vi "Robotics Environment Simulator.vi"() -> ()   [LabVIEW 2013]
doc: "This VI starts and stops the environment simulator and serves as the master VI for your simulation code. Open and run this VI to display the environment simulator, or open the block diagram to view or modify simulation code."
uses:
  <vilib>/robotics/Simulator/Engine/ctl/Step Mode.ctl
  <vilib>/robotics/Simulator/Engine/ctl/DeviceID.ctl
  <vilib>/robotics/Simulator/Engine/ctl/Robot Component ID.ctl
  <resource>/robotics/simulator/Utility/ModelBuilder/Utilities/3DController/Public/ActionType.ctl
  <resource>/robotics/simulator/Utility/ModelBuilder/Utilities/3DController/3DController.lvclass
  <instrlib>/Hitec HS400 Series/HAIOL/Hitec HS400 Series.lvclass
  <vilib>/Analysis/7linalg.llb/Real Transpose Matrix.vi
  <vilib>/Analysis/baseanly.llb/A x Vector.vi
  <vilib>/Analysis/baseanly.llb/Real A x B.vi
  <vilib>/Analysis/_algsub.llb/Real Vector Norm.vi
  <vilib>/Analysis/baseanly.llb/Outer Product.vi
  <vilib>/Analysis/baseanly.llb/Real Outer Product.vi
  <vilib>/robotics/Kinematics/Create Lie Group Matrix.vi
  <vilib>/robotics/Simulator/Interface/Simulator References/Get Robot Component Reference.vi
  <vilib>/robotics/Simulator/Interface/Simulator References/Get 3D Visual Scene Reference.vi
  <vilib>/Analysis/baseanly.llb/Real Inverse Matrix.vi
  <vilib>/Analysis/7linalg.llb/Create Special Matrix.vi
  <vilib>/Analysis/7linalg.llb/Create Special Real Matrix.vi
  <vilib>/Analysis/Matrix/Numeric/Multiply/Multiply.vi
  <vilib>/Analysis/Matrix/Numeric/Multiply/Multiply - RM,R.vi
  <vilib>/Analysis/Matrix/Numeric/Multiply/Multiply - R,RM.vi
  <vilib>/Analysis/Matrix/Numeric/Add/Add.vi
  <vilib>/Analysis/Matrix/Numeric/Add/Add - RM,RM.vi
  <vilib>/robotics/Simulator/NI_Robotics_Simulator.lvlib
  <instrlib>/Hitec HS400 Series/HAIOL/Simulator/Hitec HS400 Series Simulator.lvclass
  <resource>/objmgr/LVODE.rc
  <vilib>/Analysis/NI_AALPro.lvlib
  <vilib>/Analysis/NI_AALBase.lvlib
  <vilib>/robotics/Kinematics/NI_Kinematics.lvlib
panel:
  out "p":dbl[](array[numeric])
  out "3D Picture":refnum<vi>(3d-picture)
  out "Waveform Chart":dbl(graph)
  out "exist":bool
  out "exit":bool
  out "target pos":dbl[](array[numeric])
  out "joints":dbl[](array[numeric])
  in  "manifest filename":string="Robotics Environment Simulator.xml"
  in  "stop":bool
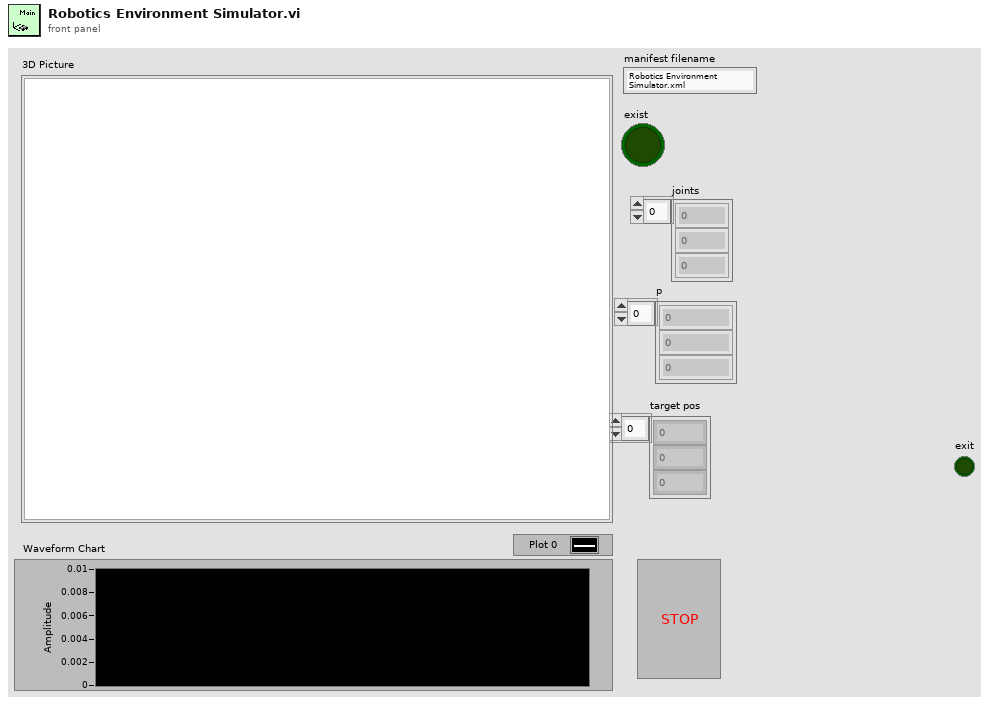
[diagram p1: front panel]
types:
  T1 = typedef "NI_Robotics_Simulator.lvlib/Step Mode.ctl" = u16
  T2 = typedef "NI_Robotics_Simulator.lvlib/DeviceID.ctl" = cluster{"robot ID":string, "sensor/actuator ID":string}
  T3 = typedef "NI_Robotics_Simulator.lvlib/Robot Component ID.ctl" = cluster{"robot ID":string, "component ID":string}
  T4 = typedef "NI_Robotics_Model_Builder.lvlib/3DController.lvclass/ActionType.ctl" = enum16{"None", "Trans_X", "Trans_Y", "Trans_Z", "Rot_X", "Rot_Y", "Rot_Z"}
  T5 = cluster{"Position[0]":sgl, "Position[1]":sgl, "Position[2]":sgl}
  T6 = typedef "NI_Matrix.lvlib/RealMatrix.ctl" = dbl[][]
  T7 = typedef "LVPoint32TypeDef.ctl" = cluster{"Horizontal":i32, "Vertical":i32}
  T8 = typedef "LV3DPointTypeDef.ctl" = cluster{"X":sgl, "Y":sgl, "Z":sgl}
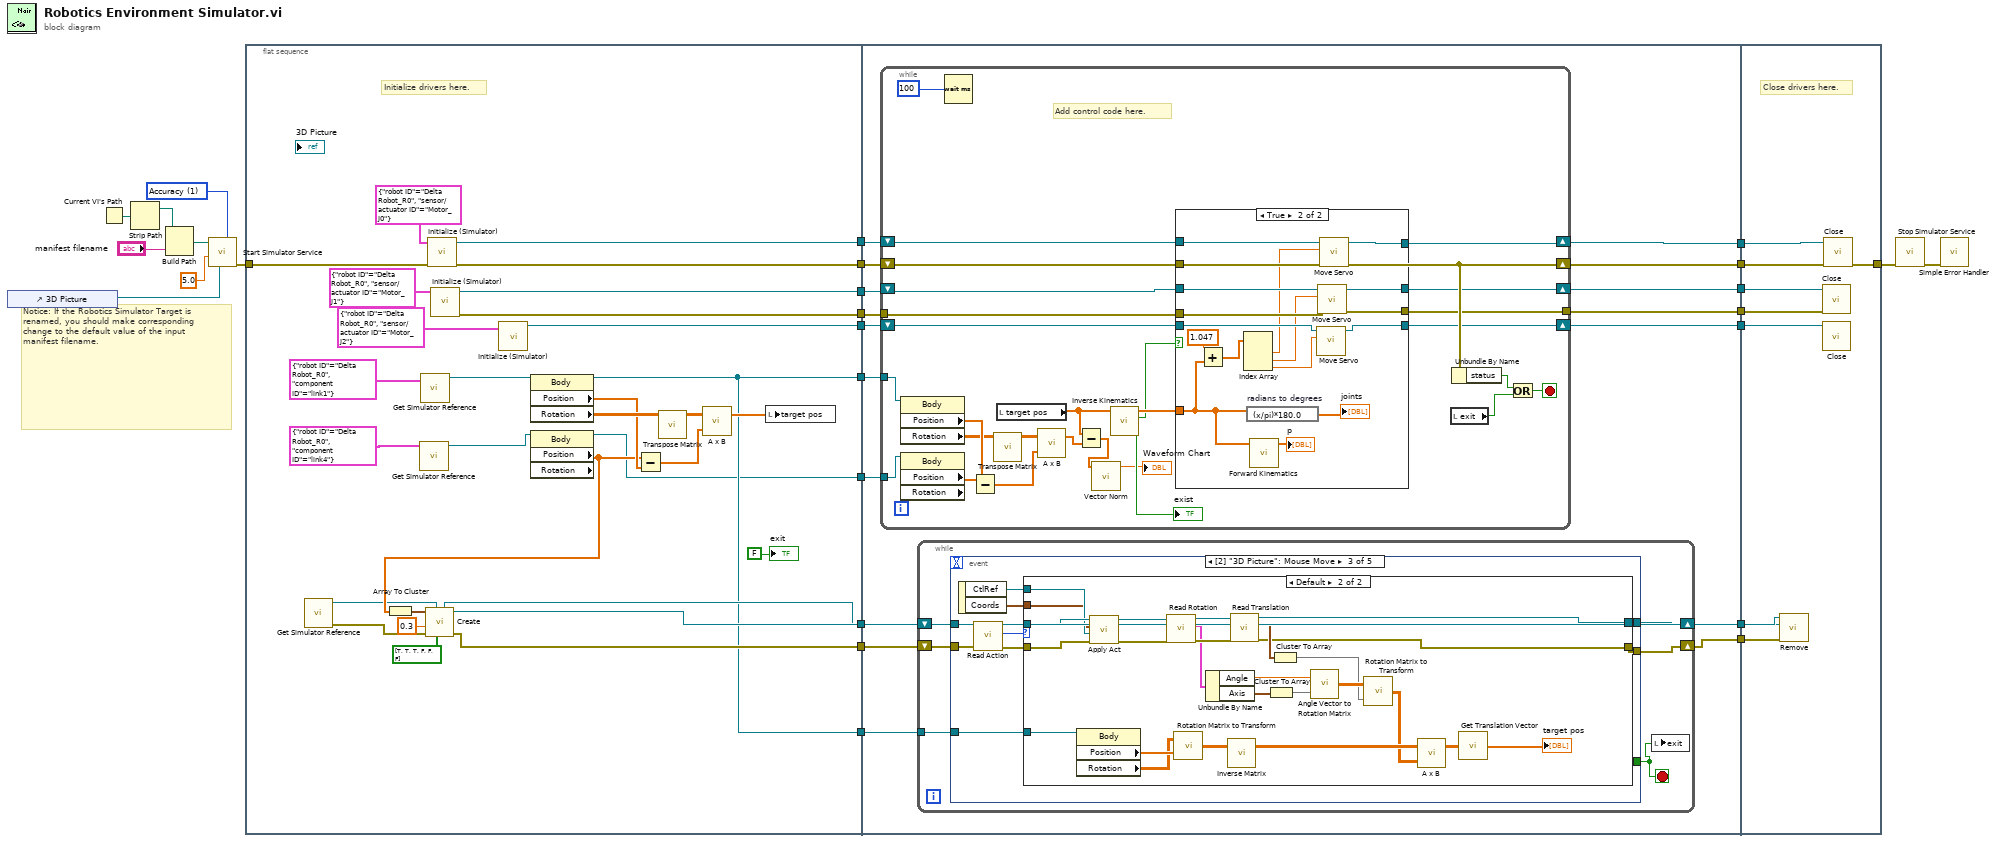
[diagram p0: block diagram]
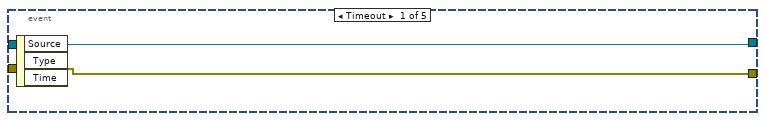
[diagram p2: hidden frame]
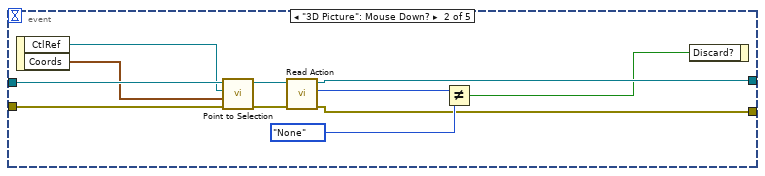
[diagram p3: hidden frame]
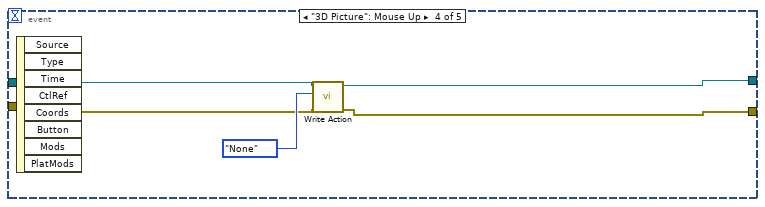
[diagram p5: hidden frame]
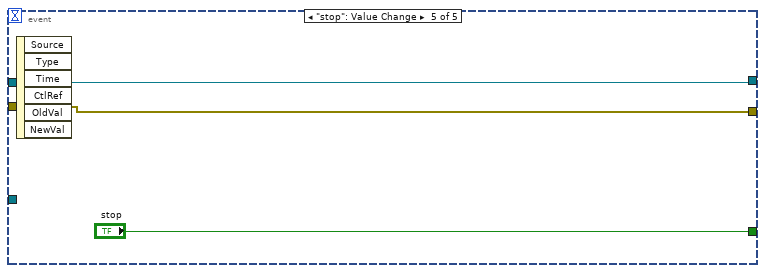
[diagram p6: hidden frame]
diagram:
  w13 = T1 1 items=["Performance", "Accuracy"] ("step mode")
  # "Notice: If the Robotics Simulator Target is renamed, you should make corresponding change to the default value of the input manifest filename."
  n1 = control-ref of="3D Picture"() -> (w1:refnum<vi>)
  n2 = Current VI's Path() -> (path=w27:path)
  n3 = Strip Path(path=w27) -> (stripped path=w26:path)  [unwired: 1 out]
  n4 = Build Path(base path=w26, name or relative path="manifest filename") -> (appended path=w25:path)
  n5 = call <vilib>:"Start Simulator Service.vi"("step mode"=w13, "3D picture refnum"=w1, "step size (ms)"=5.0 ("stepsize(ms)"), "manifest file"=w25) -> ("error out"=w22:errorcluster)  [unwired: 7 in]
  n6 = flat-sequence {
    tunnel: w22 -> [w57]
    tunnel: [w57] -> w21
    tunnel: [w56] -> w19
    tunnel: [w54] -> w17
    tunnel: [w53] -> w16
    tunnel: [w38] -> w12
    tunnel: [w37] -> w11
    tunnel: [w31] -> w10
    tunnel: [w34] -> w9
    tunnel: [w32] -> w5
    tunnel: [w31] -> w3
    tunnel: [w30] -> w2
    tunnel: w21 -> [w75]
    tunnel: [w76] -> w20
    tunnel: w19 -> [w74]
    tunnel: [w73] -> w18
    tunnel: w17 -> [w72]
    tunnel: w16 -> [w71]
    tunnel: [w70] -> w15
    tunnel: [w69] -> w14
    tunnel: w12 -> [w68]
    tunnel: w11 -> [w67]
    tunnel: w10 -> [w66]
    tunnel: w9 -> [w65]
    tunnel: [w64] -> w8
    tunnel: [w63] -> w7
    tunnel: [w62] -> w6
    tunnel: w5 -> [w61]
    tunnel: [w61] -> w4
    tunnel: w3 -> [w60]
    tunnel: w2 -> [w59]
    tunnel: [w194] -> w28
    tunnel: w20 -> [w196]
    tunnel: w18 -> [w195]
    tunnel: w15 -> [w193]
    tunnel: w14 -> [w192]
    tunnel: w8 -> [w191]
    tunnel: w7 -> [w190]
    tunnel: w6 -> [w189]
    tunnel: w4 -> [w188]
    frame #0 {
      # "Initialize drivers here."
      n7 = call-poly <vilib>:"Get Simulator Reference.vi"() -> ("error out"=w40:errorcluster, "scene ref"=w41:refnum<vi>)  [unwired: 10 in]
      n8 = call-poly <vilib>:"Get Simulator Reference.vi"("robot component ID"=T3 {"robot ID"="Delta Robot_R0", "component ID"="link4"}) -> ("component ref"=w44:refnum<k20>)  [unwired: 9 in, 1 out]
      n9 = call-poly <vilib>:"Get Simulator Reference.vi"("robot component ID"=T3 {"robot ID"="Delta Robot_R0", "component ID"="link1"}) -> ("component ref"=w45:refnum<k20>)  [unwired: 9 in, 1 out]
      n10 = call <instrlib>:"Initialize (Simulator).vi"("error in (no error)"=w57, "Device ID"=T2 {"robot ID"="Delta Robot_R0", "sensor/actuator ID"="Motor_J0"}) -> ("Hitec HS400 Series out"=w56:refnum<class "Hitec HS400 Series.lvclass">)  [unwired: 8 in, 1 out]
      n11 = call <instrlib>:"Initialize (Simulator).vi"("Device ID"=T2 {"robot ID"="Delta Robot_R0", "sensor/actuator ID"="Motor_J1"}) -> ("error out"=w53:errorcluster, "Hitec HS400 Series out"=w54:refnum<class "Hitec HS400 Series.lvclass">)  [unwired: 9 in]
      n12 = call <instrlib>:"Initialize (Simulator).vi"("Device ID"=T2 {"robot ID"="Delta Robot_R0", "sensor/actuator ID"="Motor_J2"}) -> ("Hitec HS400 Series out"=w34:refnum<class "Hitec HS400 Series.lvclass">)  [unwired: 9 in, 1 out]
      n13 = property class="Body"(reference=w45) -> (reference out=w31:refnum<k20>, "Position"=w46:sgl[], "Rotation"=w47:sgl[][])  [unwired: 1 in, 1 out]
      n14 = property class="Body" props=["Position", "Rotation"](reference=w44) -> (reference out=w30:refnum<k20>, "Position"=w42:sgl[])  [unwired: 1 in, 2 out]
      n15 = Array To Cluster(array=w42) -> (cluster=w43:T5)
      n16 = call <resource>:"Create.vi"("Marks"=bool[] [TRUE, TRUE, TRUE, FALSE, FALSE, FALSE], "Model Root"=w41, "error in (no error)"=w40, "Scale"=0.3, "Translation"=w43) -> ("error out"=w37:errorcluster, "3DController"=w38:refnum<class "3DController.lvclass">, "Model Root out"=w32:refnum<vi>)  [unwired: 4 in]
      n17 = Subtract(x=w42, y=w46) -> (x-y=w49:sgl[])
      n18 = call-poly <vilib>:"Transpose Matrix.vi"("Input Matrix"=w47) -> ("Matrix Transpose"=w48:T6)  [unwired: 9 in, 1 out]
      n19 = call-poly <vilib>:"A x B.vi"("Vector"=w49, "A"=w48) -> ("A x Vector"=w36:dbl[])  [unwired: 1 out]
      n20 = local write "target pos"(w36) -> ()
      "exit" <- FALSE ("exit")
    }
    frame #1 {
      n21 = while {
        shift-right: [w166] -> w76
        shift-left: w75 -> [w166]
        shift-right: [w163] -> w73
        shift-left: w74 -> [w164]
        tunnel: w71 -> [w161]
        tunnel: [w160] -> w70
        shift-right: [w159] -> w69
        shift-left: w72 -> [w162]
        shift-right: [w157] -> w64
        shift-left: w65 -> [w158]
        tunnel: w60 -> [w146]
        tunnel: w59 -> [w145]
        stop <- w152 stop-if-true
        # "Add control code here."
        n22 = property class="Body"(reference=w146) -> ("Position"=w150:sgl[], "Rotation"=w149:sgl[][])  [unwired: 1 in, 2 out]
        n23 = property class="Body" props=["Position", "Rotation"](reference=w145) -> ("Position"=w151:sgl[])  [unwired: 1 in, 3 out]
        n24 = Wait (ms)(milliseconds to wait=100) -> ()  [unwired: 1 out]
        n25 = Subtract(x=w151, y=w150) -> (x-y=w147:sgl[])
        n26 = call-poly <vilib>:"Transpose Matrix.vi"("Input Matrix"=w149) -> ("Matrix Transpose"=w148:T6)  [unwired: 9 in, 1 out]
        n27 = local read "target pos"() -> (w144:dbl[])
        n28 = call-poly <vilib>:"A x B.vi"("Vector"=w147, "A"=w148) -> ("A x Vector"=w143:dbl[])  [unwired: 1 out]
        n29 = Subtract(x=w144, y=w143) -> (x-y=w142:dbl[])
        n30 = call-poly <vilib>:"Vector Norm.vi"("Input Vector"=w142) -> ("norm"=→"Waveform Chart":dbl)  [unwired: 9 in, 1 out]
        n31 = call "Inverse Kinematics.vi"("p"=w144) -> ("exist"=w155:bool, "joints"=w156:dbl[])  [unwired: 9 in]
        "exist" <- w155
        n32 = case shown="True" w155 {
          tunnel: w166 -> [_ w187]
          tunnel: w164 -> [w170 w186]
          tunnel: [w170 w185] -> w163
          tunnel: w162 -> [w169 w184]
          tunnel: w161 -> [w168 w183]
          tunnel: [w168 w182] -> w160
          tunnel: [w169 w181] -> w159
          tunnel: w156 -> [_ w172]
          tunnel: w158 -> [w167 w179]
          tunnel: [w167 w178] -> w157
          frame False {
          }
          frame True {
            n33 = Add(x=1.047, y=w172) -> (x+y=w174:dbl[])
            n34 = Index Array(array=w174) -> (element #1=w177:dbl, element #2=w176:dbl, element #3=w175:dbl)  [unwired: 3 in]
            n35 = expression code="(x/pi)*180.0" "radians to degrees"(w172) -> (→"joints":dbl[])
            n36 = call "Forward Kinematics.vi"("joints"=w172) -> ("p"=→"p":dbl[])  [unwired: 9 in, 1 out]
            n37 = call-dynamic "Move Servo.vi"("CCW Position (0.0 rad)"=w175, "Hitec HS400 Series in"=w179) -> ("Hitec HS400 Series out"=w178:refnum<class "Hitec HS400 Series.lvclass">)  [unwired: 8 in, 1 out]
            n38 = call-dynamic "Move Servo.vi"("error in (no error)"=w183, "CCW Position (0.0 rad)"=w176, "Hitec HS400 Series in"=w184) -> ("error out"=w182:errorcluster, "Hitec HS400 Series out"=w181:refnum<class "Hitec HS400 Series.lvclass">)  [unwired: 7 in]
            n39 = call-dynamic "Move Servo.vi"("error in (no error)"=w187, "CCW Position (0.0 rad)"=w177, "Hitec HS400 Series in"=w186) -> ("Hitec HS400 Series out"=w185:refnum<class "Hitec HS400 Series.lvclass">)  [unwired: 7 in, 1 out]
          }
        }
        n40 = local read "exit"() -> (w153:bool)
        n41 = Unbundle By Name(w166) -> ("status"=w165:bool)
        n42 = Or(x=w165, y=w153) -> (x .or. y?=w152:bool)
      }
      n43 = while {
        shift-right: [w80] -> w62
        shift-left: w68 -> [w82]
        shift-right: [w79] -> w63
        shift-left: w67 -> [w81]
        tunnel: w66 -> [w78]
        stop <- w77 stop-if-true
        n44 = event shown="[2] \"3D Picture\": Mouse Move" {
          selector: _ -> [_ _ _ _ _]
          dyn-events: _ -> [_ _ _ _ _]
          timeout: _ -> [_ _ _ _ _]
          tunnel: w82 -> [w84 w91 w105 w136 w140]
          tunnel: w81 -> [w83 w90 w104 w135 w139]
          tunnel: [w84 w87 w97 w134 w140] -> w80
          tunnel: [w83 w86 w96 w133 w139] -> w79
          tunnel: w78 -> [_ _ w98 _ _]
          tunnel: [_ _ _ _ "stop"] -> w77
          event Timeout {
            n45 = event-data() -> ()  [unwired: 1 in, 3 out]
          }
          event "3D Picture": Mouse Down? {
            n46 = event-data() -> ("CtlRef"=w89:refnum<vi>, "Coords"=w88:T7)  [unwired: 1 in]
            n47 = call-dynamic "Point to Selection.vi"("error in (no error)"=w90, "Coords"=w88, "CtlRef"=w89, "3DController in"=w91) -> ("error out"=w95:errorcluster, "3DController out"=w94:refnum<class "3DController.lvclass">)  [unwired: 6 in]
            n48 = call-dynamic "Read Action.vi"("error in (no error)"=w95, "3DController in"=w94) -> ("error out"=w86:errorcluster, "Action"=w93:T4, "3DController out"=w87:refnum<class "3DController.lvclass">)  [unwired: 7 in]
            n49 = Not Equal?(x=w93, y=ActionType."None") -> (x != y?=w85:bool)
            n50 = event-data("Discard?"=w85) -> ()  [unwired: 1 in, 1 out]
          }
          event "3D Picture": Mouse Move {
            n51 = event-data() -> ("CtlRef"=w100:refnum<vi>, "Coords"=w99:T7)  [unwired: 1 in]
            n52 = call-dynamic "Read Action.vi"("error in (no error)"=w104, "3DController in"=w105) -> ("error out"=w101:errorcluster, "Action"=w103:T4, "3DController out"=w102:refnum<class "3DController.lvclass">)  [unwired: 7 in]
            n53 = case shown="Default" w103 {
              tunnel: w102 -> [w107 w116]
              tunnel: w101 -> [w106 w115]
              tunnel: w100 -> [_ w114]
              tunnel: w99 -> [_ w113]
              tunnel: w98 -> [_ w112]
              tunnel: [w107 w109] -> w97
              tunnel: [w106 w108] -> w96
              frame "None" {
              }
              frame Default {
                n54 = property class="Body"(reference=w112) -> ("Position"=w121:sgl[], "Rotation"=w120:sgl[][])  [unwired: 1 in, 2 out]
                n55 = call-dynamic "Apply Act.vi"("error in (no error)"=w115, "3D Scene"=w114, "End Point"=w113, "3DController in"=w116) -> ("error out"=w131:errorcluster, "3DController out"=w132:refnum<class "3DController.lvclass">)  [unwired: 6 in]
                n56 = call-dynamic "Read Rotation.vi"("error in (no error)"=w131, "3DController in"=w132) -> ("error out"=w129:errorcluster, "Rotation"=w128:cluster{"Axis":T8, "Angle":sgl}, "3DController out"=w130:refnum<class "3DController.lvclass">)  [unwired: 7 in]
                n57 = call <vilib>:"Rotation Matrix to Transform.vi"("translation vector"=w121, "rotation matrix"=w120) -> ("transform"=w119:T6)
                n58 = Unbundle By Name(w128) -> ("Angle"=w125:sgl, "Axis"=w127:T8)
                n59 = call-poly <vilib>:"Inverse Matrix.vi"("Input Matrix"=w119) -> ("Inverse Matrix"=w118:T6)  [unwired: 1 in, 1 out]
                n60 = call-dynamic "Read Translation.vi"("error in (no error)"=w129, "3DController in"=w130) -> ("error out"=w108:errorcluster, "3D Point"=w123:T8, "3DController out"=w109:refnum<class "3DController.lvclass">)  [unwired: 7 in]
                n61 = Cluster To Array(cluster=w127) -> (array=w126:sgl[])
                n62 = Cluster To Array(cluster=w123) -> (array=w122:sgl[])
                n63 = call <vilib>:"Angle Vector to Rotation Matrix.vi"("vector"=w126, "angle"=w125) -> ("rotation matrix"=w124:T6)
                n64 = call <vilib>:"Rotation Matrix to Transform.vi"("translation vector"=w122, "rotation matrix"=w124) -> ("transform"=w117:T6)
                n65 = call-poly <vilib>:"A x B.vi"("B"=w117, "A"=w118) -> ("A x B"=w111:T6)  [unwired: 1 out]
                n66 = call <vilib>:"Get Translation Vector.vi"("transform"=w111) -> ("translation vector"=→"target pos":dbl[])
              }
            }
          }
          event "3D Picture": Mouse Up {
            n67 = event-data() -> ()  [unwired: 1 in, 8 out]
            n68 = call-dynamic "Write Action.vi"("error in (no error)"=w135, "Action"=ActionType."None", "3DController in"=w136) -> ("error out"=w133:errorcluster, "3DController out"=w134:refnum<class "3DController.lvclass">)  [unwired: 7 in]
          }
          event "stop": Value Change {
            n69 = event-data() -> ()  [unwired: 1 in, 6 out]
          }
        }
        n70 = local write "exit"(w77) -> ()
      }
    }
    frame #2 {
      # "Close drivers here."
      n71 = call-dynamic "Remove.vi"("error in (no error)"=w190, "Model Root"=w188, "3DController in"=w189) -> ()  [unwired: 7 in, 2 out]
      n72 = call-dynamic "Close.vi"("error in (no error)"=w193, "Hitec HS400 Series in"=w192) -> ()  [unwired: 9 in, 1 out]
      n73 = call-dynamic "Close.vi"("Hitec HS400 Series in"=w191) -> ()  [unwired: 10 in, 1 out]
      n74 = call-dynamic "Close.vi"("error in (no error)"=w196, "Hitec HS400 Series in"=w195) -> ("error out"=w194:errorcluster)  [unwired: 9 in]
    }
  }
  n75 = call <vilib>:"Stop Simulator Service.vi"("error in (no error)"=w28) -> ("error out"=w23:errorcluster)  [unwired: 10 in]
  n76 = call <vilib>:"Simple Error Handler.vi"("error in (no error)"=w23) -> ()  [unwired: 4 in, 5 out]
